vi "Send Unsubscribe.vi"(7 "Message Priority (High)":T1=enum."High", 8 "error in (no error)":errorcluster, 9 "Data Array":refnum<class "Data.lvclass">[](array[class]), 10 "Message Array":refnum<class "Message.lvclass">[](array[class]), 11 "Actor in":refnum<class "Actor.lvclass">) -> (0 "error out":errorcluster, 3 "Actor out":refnum<class "Actor.lvclass">)   [LabVIEW 2020, in "Publisher.lvlib" / "Unsubscribe Msg.lvclass"]
doc: "This VI sends the message to an actor."
uses:
  Unsubscribe Msg.lvclass
  PPL/HDH.Actor Framework.Core.Actor.lvlibp/1abvi3w/vi.lib/ActorFramework/Actor/Actor.lvclass
  PPL/HDH.Actor Framework.Core.Actor.lvlibp/1abvi3w/vi.lib/ActorFramework/Message Enqueuer/Message Priority.ctl
  PPL/HDH.Actor Framework.Core.Actor.lvlibp/1abvi3w/vi.lib/ActorFramework/Message/Message.lvclass
  PPL/HDH.Data.Generic.lvlibp/Data.lvclass
  C:/Current projects/WS/HDH.ActorFramework.Core/Actor/Publisher/Publisher Messages/Publisher Msg/Publisher Msg.lvclass
  Unsubscribe Msg.lvclass/Unsubscribe Msg.ctl
  Publisher Msg/Publisher Msg.lvclass
  PPL/HDH.Actor Framework.Core.Utility.lvlibp
  PPL/HDH.Actor Framework.Core.Actor.lvlibp/1abvi3w/vi.lib/ActorFramework/Message Enqueuer/Message Enqueuer.lvclass
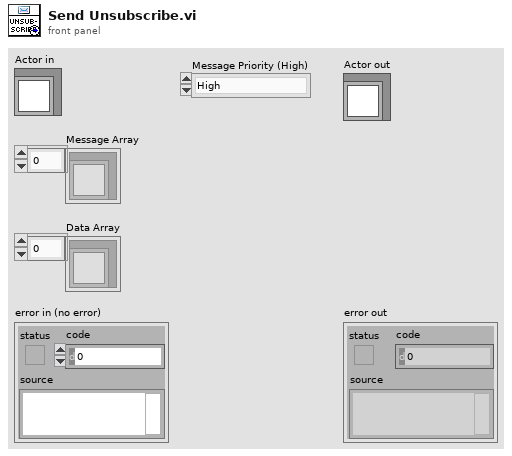
[diagram p1: front panel]
types:
  T1 = typedef "HDH.Actor Framework.Core.Actor.lvlibp/Message Enqueuer.lvclass/Message Priority.ctl" = enum16{"Low", "Normal", "High"}
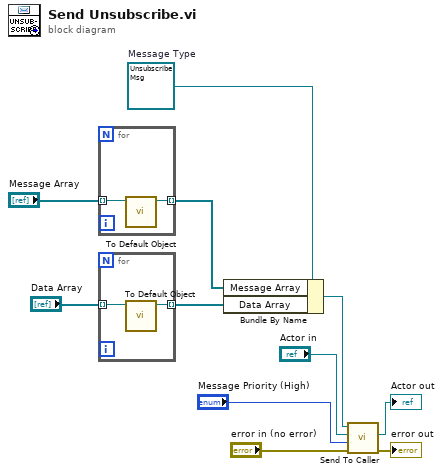
[diagram p0: block diagram]
diagram:
  w11 = refnum<class "Unsubscribe Msg.lvclass"> refnum  # Message Type
  n1 = for {
    tunnel: "Message Array" -> [w13] mode=indexing
    tunnel: [w12] -> w3 mode=indexing
    n2 = call "To Default Object.vi"("Object in"=w13) -> ("Default out"=w12:refnum<class "Message.lvclass">)  [unwired: 10 in]
  }
  n3 = for {
    tunnel: "Data Array" -> [w15] mode=indexing
    tunnel: [w14] -> w1 mode=indexing
    n4 = call "To Default Object.vi"("Object in"=w15) -> ("Default out"=w14:refnum<class "Data.lvclass">)  [unwired: 10 in]
  }
  n5 = Bundle By Name(cluster=w11, "Message Array"=w3, "Data Array"=w1) -> (w5:refnum<class "Unsubscribe Msg.lvclass">)
  n6 = call "Send To Caller.vi"("error in (no error)"="error in (no error)", "Message Priority (Normal)"="Message Priority (High)", "Actor in"="Actor in", "Publisher Msg in"=w5) -> ("error out"=→"error out":errorcluster, "Actor out"=→"Actor out":refnum<class "Actor.lvclass">)  [unwired: 5 in, 1 out]
